vi "ReadTemperature.vi"(0 "object in":refnum<class "TC0608.lvclass">, 5 "error in (no error)":errorcluster) -> (14 "object out":refnum<class "TC0608.lvclass">, 16 "temperature (C)":dbl, 19 "error out":errorcluster)   [LabVIEW 2023, in "TC0608.lvclass"]
uses:
  TC0608.lvclass
  TC0608.lvclass/TC0608.ctl
  Peltier controller TC/TCxxxx/TCxxxx.lvlib
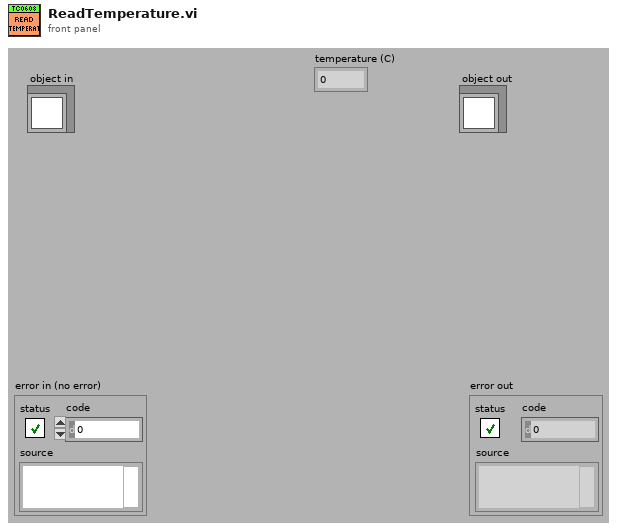
[diagram p1: front panel]
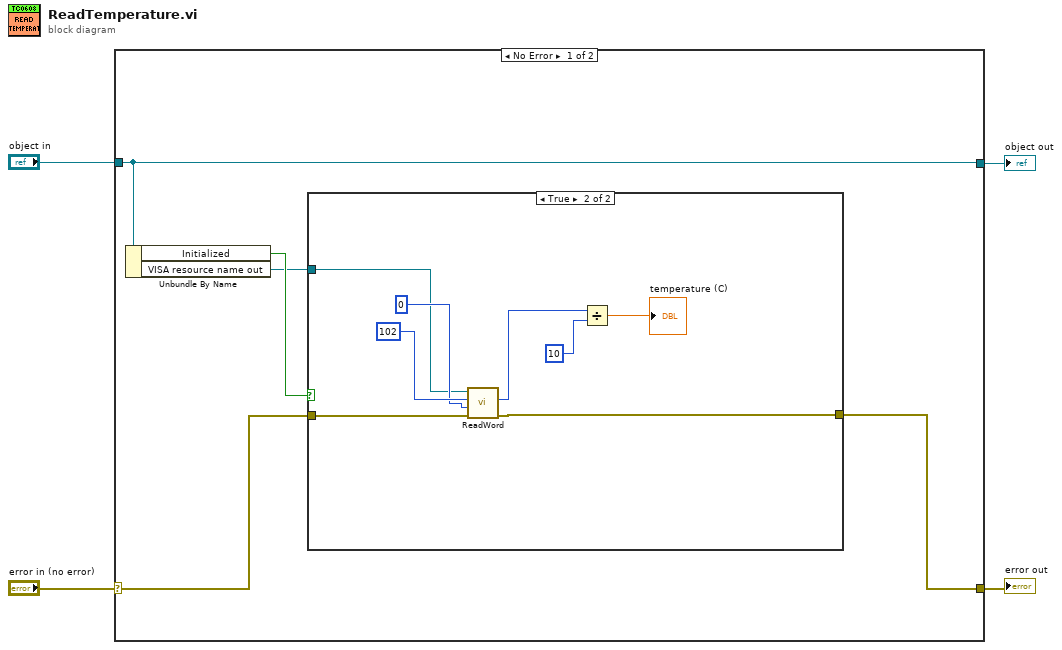
[diagram p0: block diagram]
diagram:
  n1 = case shown="No Error" "error in (no error)" {
    selector: "error in (no error)" -> [w6 w20]
    tunnel: [w5 w20] -> w3
    tunnel: [w9 w19] -> w1
    tunnel: "object in" -> [w9 w19]
    frame No Error {
      n2 = Unbundle By Name(w9) -> ("Initialized"=w8:bool, "VISA resource name out"=w7:refnum<visa-resource-name>)
      n3 = case shown="True" w8 {
        tunnel: w7 -> [_ w13]
        tunnel: w6 -> [w10 w12]
        tunnel: [w10 w11] -> w5
        frame False {
        }
        frame True {
          n4 = call "ReadWord.vi"("error in (no error)"=w12, "Parameter [0 ... 65535]"=u16 0, "Befehl [0 ... 65535]"=u16 102, "VISA resource name"=w13) -> ("error out"=w11:errorcluster, "Regler Rückgabewert [0 ... 65535]"=w16:u16)  [unwired: 4 in, 2 out]
          n5 = Divide(x=w16, y=u16 10) -> (x/y=→"temperature (C)":dbl)
        }
      }
    }
    frame Error {
    }
  }
  "error out" <- w3
  "object out" <- w1
